vi "Disconnect.vi"(8 "error in (no error)":errorcluster, 11 "EPU452 in":refnum<class "EPU452.lvclass">) -> (0 "error out":errorcluster)   [LabVIEW 2018, in "EPU452.lvclass"]
uses:
  EPU452.lvclass
  <vilib>/Instr/_visa.llb/VISA Flush IO Buffer Mask.ctl
  EPU452.lvclass/EPU452.ctl
panel:
  out "EPU452 out":refnum<class "EPU452.lvclass">
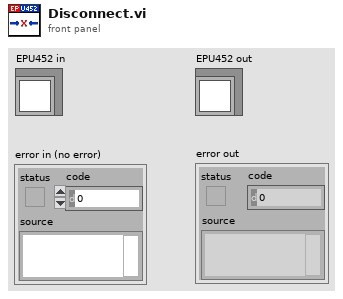
[diagram p1: front panel]
types:
  T1 = typedef "VISA Flush IO Buffer Mask.ctl" = u16
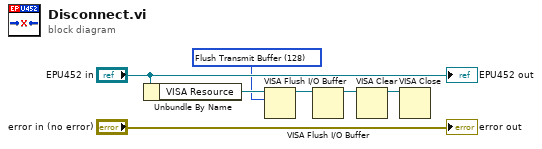
[diagram p0: block diagram]
diagram:
  w1 = T1 128 items=["Flush Receive Buffer"=16, "Write Transmit Buffer to Device"=32, "Flush Receive Buffer (No I/O)"=64, "Flush Transmit Buffer"=128] ("Mask")
  n1 = Unbundle By Name("EPU452 in") -> ("VISA Resource"=w3:refnum<visa-resource-name>)
  n2 = VISA Flush I/O Buffer(VISA resource name=w3, mask (16)=w1) -> (VISA resource name out=w2:refnum<visa-resource-name>)  [unwired: 1 in, 1 out]
  n3 = VISA Flush I/O Buffer(VISA resource name=w2) -> (VISA resource name out=w4:refnum<visa-resource-name>)  [unwired: 2 in, 1 out]
  n4 = VISA Clear(VISA resource name=w4) -> (VISA resource name out=w5:refnum<visa-resource-name>)  [unwired: 1 in, 1 out]
  n5 = VISA Close(VISA resource name=w5) -> ()  [unwired: 1 in, 1 out]
  "error out" <- "error in (no error)"
  "EPU452 out" <- "EPU452 in"
